vi "get_current_selection.vi"(8 "error in":errorcluster, 11 "vs_tree_control in":refnum<class "vs_tree_control.lvclass">) -> (0 "error out":errorcluster, 1 "Selection ID":u64, 2 "Selection Reference":refnum<k24>, 3 "vs_tree_control out":refnum<class "vs_tree_control.lvclass">, 4 "Selection Name":string)   [LabVIEW 2020, in "vs_tree_control.lvclass"]
uses:
  vs_tree_control.lvclass
  NationalInstruments.VeriStand.SystemStorage
  vs_tree_control.lvclass/vs_tree_control.ctl
  NationalInstruments.VeriStand.SystemStorageUI
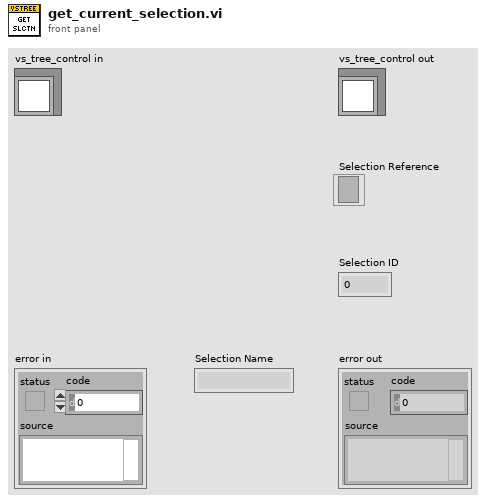
[diagram p1: front panel]
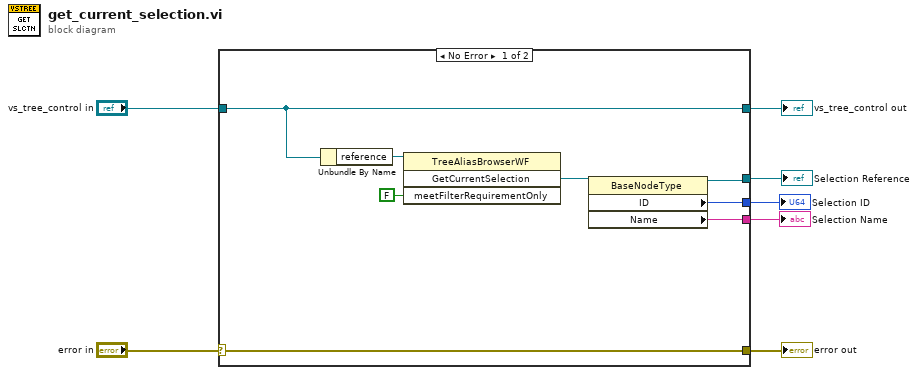
[diagram p0: block diagram]
diagram:
  n1 = case shown="No Error" "error in" {
    selector: "error in" -> [w15 w17]
    tunnel: [w15 w17] -> w6
    tunnel: [w14 w16] -> w4
    tunnel: "vs_tree_control in" -> [w14 w16]
    tunnel: [w10 _] -> w3
    tunnel: [w9 _] -> w2
    tunnel: [w8 _] -> w1
    frame No Error {
      n2 = Unbundle By Name(w14) -> ("reference"=w13:refnum<k24>)
      n3 = invoke class="TreeAliasBrowserWF" method="GetCurrentSelection"(reference=w13, "meetFilterRequirementOnly"=FALSE) -> ("GetCurrentSelection"=w11:refnum<k24>)  [unwired: 2 in, 3 out]
      n4 = property class="BaseNodeType"(reference=w11) -> (reference out=w10:refnum<k24>, "ID"=w9:u64, "Name"=w8:string)  [unwired: 1 in, 1 out]
    }
    frame Error {
    }
  }
  "error out" <- w6
  "vs_tree_control out" <- w4
  "Selection Reference" <- w3
  "Selection ID" <- w2
  "Selection Name" <- w1
